vi "Initialize_Power_Meter.vi"(8 "error in (no error)":errorcluster, 11 "VISA Refnum in":refnum<visa-resource-name>="PWR_SENSOR") -> (0 "error out":errorcluster)   [LabVIEW 2015]
uses:
  <instrlib>/Agilent U2000 Series/Agilent U2000 Series.lvlib
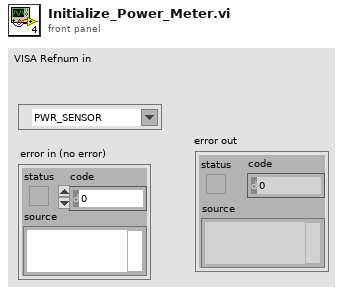
[diagram p1: front panel]
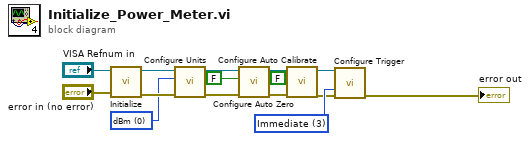
[diagram p0: block diagram]
diagram:
  w9 = u16 0 items=["dBm", "W"] ("Units")
  w14 = 3 items=["Bus", "External", "Hold", "Immediate", "Internal A"] ("Trigger Source (3: Immediate)")
  n1 = call <instrlib>:"Initialize.vi"("error in (no error)"="error in (no error)", "VISA resource name"="VISA Refnum in") -> ("error out"=w10:errorcluster, "VISA resource name out"=w11:refnum<visa-resource-name>)  [unwired: 2 in, 6 out]
  n2 = call <instrlib>:"Configure Units.vi"("error in (no error)"=w10, "Units (0: dBm)"=w9, "VISA resource name"=w11) -> ("error out"=w8:errorcluster, "VISA resource name out"=w7:refnum<visa-resource-name>)  [unwired: 1 in, 6 out]
  n3 = call <instrlib>:"Configure Auto Zero.vi"("error in (no error)"=w8, "Auto Zero (T: Enable)"=FALSE, "VISA resource name"=w7) -> ("error out"=w5:errorcluster, "VISA resource name out"=w4:refnum<visa-resource-name>)  [unwired: 7 in]
  n4 = call <instrlib>:"Configure Auto Calibrate.vi"("error in (no error)"=w5, "Auto Calibrate (T: Enable)"=FALSE, "VISA resource name"=w4) -> ("error out"=w13:errorcluster, "VISA resource name out"=w12:refnum<visa-resource-name>)  [unwired: 7 in]
  n5 = call <instrlib>:"Configure Trigger.vi"("VISA resource name"=w12, "Trigger Source (3: Immediate)"=w14, "error in (no error)"=w13) -> ("error out"=→"error out":errorcluster)  [unwired: 11 in, 1 out]
